vi "Calculate CRC.vi"(11 "data":u8[](array[numeric])) -> (3 "CRC-16":u16)   [LabVIEW 2013, in "Modbus Library - Advance.lvlib" / "RTU Data Unit.lvclass"]
doc: "Performs a cyclic redundancy check."
uses:
  RTU Data Unit.lvclass
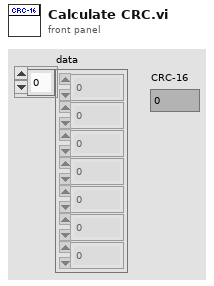
[diagram p1: front panel]
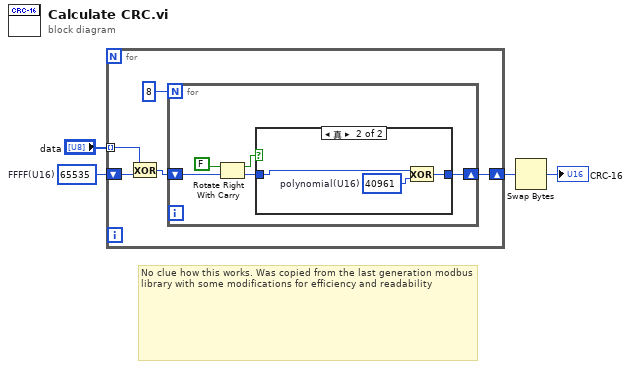
[diagram p0: block diagram]
diagram:
  w4 = u16 65535  # FFFF(U16)
  # "No clue how this works. Was copied from the last generation modbus library with some modifications for efficiency and readability"
  n1 = for {
    tunnel: "data" -> [w9] mode=indexing
    shift-right: [w6] -> w3
    shift-left: w4 -> [w8]
    n2 = Exclusive Or(1:w8, 2:w9) -> (0:w7:u16)
    n3 = for {
      N: 8 -> [_]
      shift-right: [w11] -> w6
      shift-left: w7 -> [w10]
      n4 = Rotate Right With Carry(2:w10, 3:FALSE) -> (0:w12:u16, 1:w13:bool)
      n5 = case shown="真" w13 {
        tunnel: w12 -> [w15 w18]
        tunnel: [w15 w16] -> w11
        frame False {
        }
        frame True {
          w17 = u16 40961  # polynomial(U16)
          n6 = Exclusive Or(1:w17, 2:w18) -> (0:w16:u16)
        }
      }
    }
  }
  n7 = Swap Bytes(anything=w3) -> (byte swapped=→"CRC-16":u16)
